vi "Write DVR.vi"(8 "error in (no error)":errorcluster, 10 "DVR":refnum<data-value>, 11 "Time Protocol in":refnum<class "Time Protocol.lvclass">) -> (0 "error out":errorcluster, 3 "Time Protocol out":refnum<class "Time Protocol.lvclass">)   [LabVIEW 2012, in "Time Protocol Actor.lvlib" / "Time Protocol.lvclass"]
uses:
  Time Protocol.lvclass
  Time Protocol.lvclass/Time Protocol.ctl
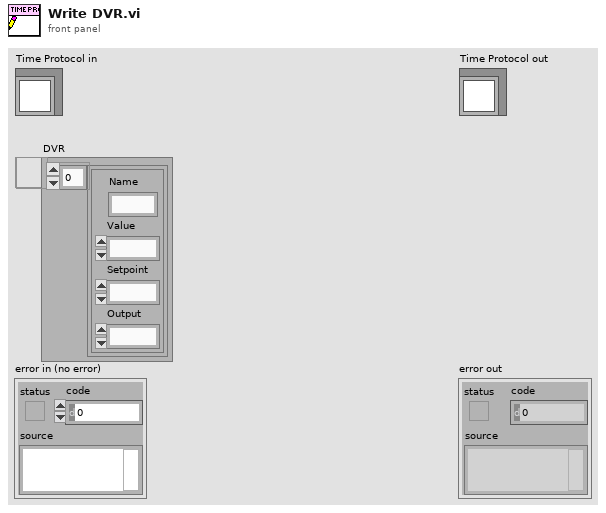
[diagram p1: front panel]
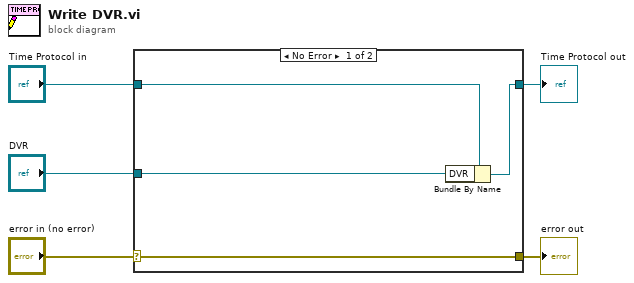
[diagram p0: block diagram]
diagram:
  n1 = case shown="No Error" "error in (no error)" {
    selector: "error in (no error)" -> [w9 w10]
    tunnel: [w9 w10] -> w4
    tunnel: [w7 w11] -> w2
    tunnel: "Time Protocol in" -> [w8 w11]
    tunnel: "DVR" -> [w6 _]
    frame No Error {
      n2 = Bundle By Name(cluster=w8, "DVR"=w6) -> (w7:refnum<class "Time Protocol.lvclass">)
    }
    frame Error {
    }
  }
  "error out" <- w4
  "Time Protocol out" <- w2
